vi "Field Draw Robots.vi"(3 "Draw Targets?":T1, 4 "RobotRef":refnum<class "Robot.lvclass">[](array[class]), 5 "Draw Number":bool=TRUE, 6 "color(black)":u32, 8 "Picture In":picture, 9 "Offset":cluster{"Width":dbl, "Height":dbl}, 10 "Scale":dbl, 11 "color":enum16{"Azul", "Amarelo"}(ring)) -> (0 "Picture Out":picture, 1 "Offset Out":cluster{"Width":dbl, "Height":dbl}, 2 "Scale Out":dbl)   [LabVIEW 2018]
uses:
  DrawTargets.ctl
  Robot_class/Robot.lvclass
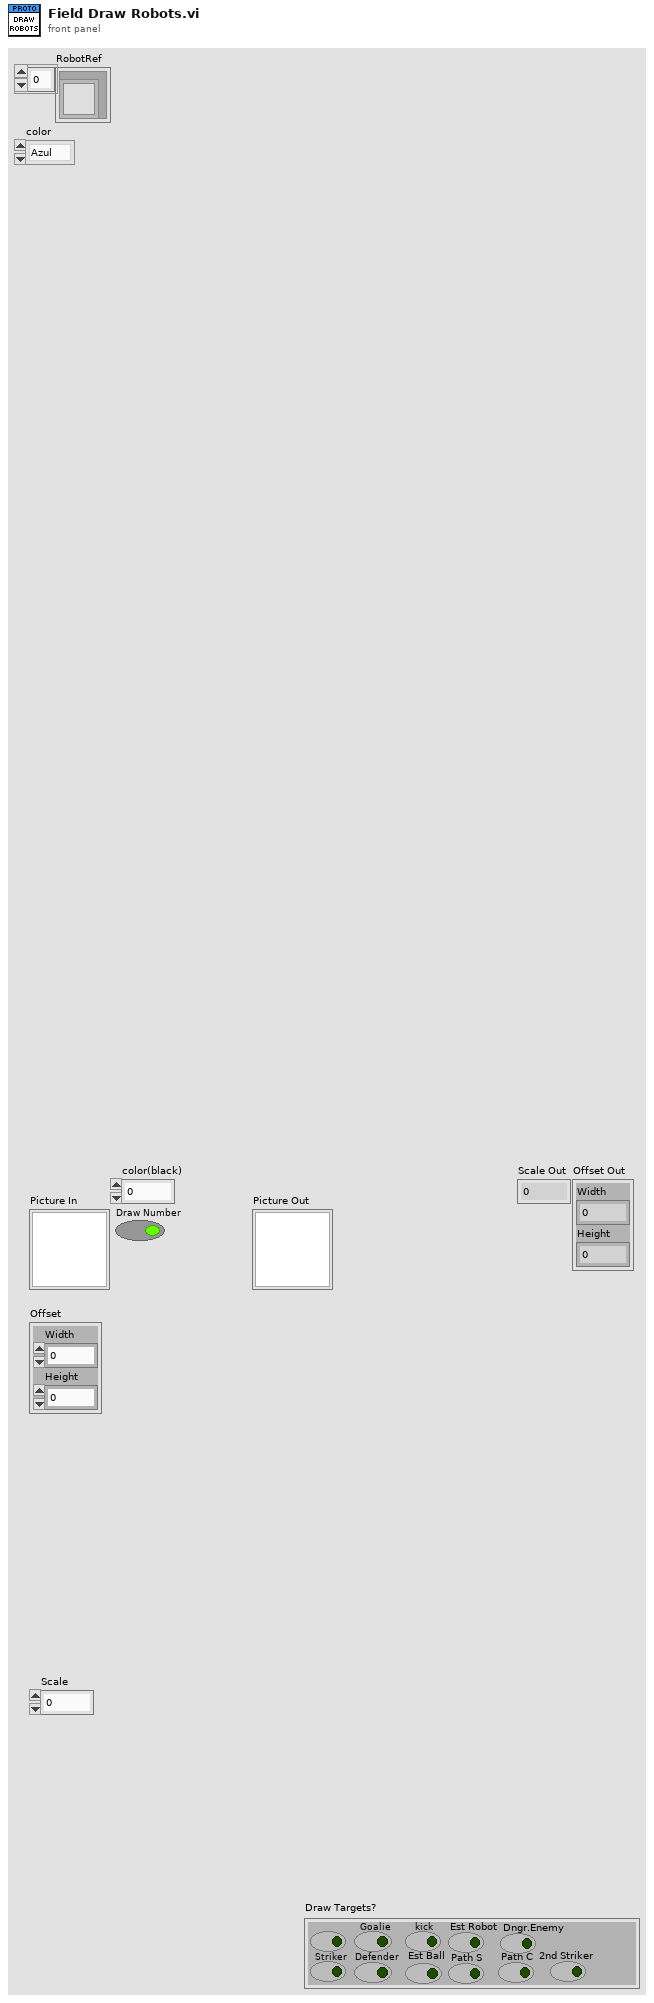
[diagram p1: front panel]
types:
  T1 = typedef "DrawTargets.ctl" = cluster{"Attacker":bool, "Striker":bool, "Goalie":bool, "Defender":bool, "kick":bool, "Est Ball":bool, "Est Robot":bool, "Path S":bool, "Path C":bool, "Dngr.Enemy":bool, "2nd Striker":bool}
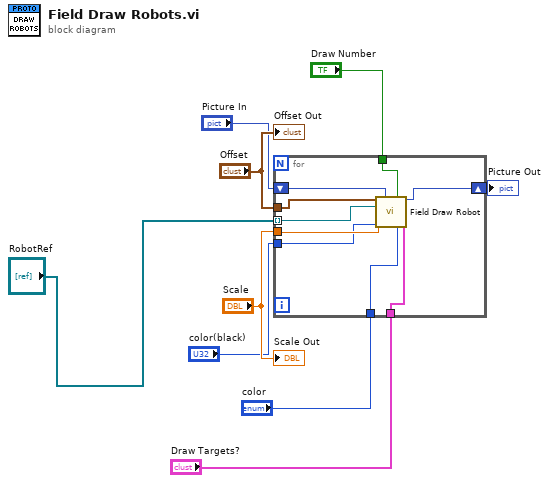
[diagram p0: block diagram]
diagram:
  n1 = for {
    tunnel: "Scale" -> [w14]
    tunnel: "Offset" -> [w15]
    shift-right: [w18] -> w5
    shift-left: "Picture In" -> [w16]
    tunnel: "color(black)" -> [w13]
    tunnel: "Draw Number" -> [w17]
    tunnel: "Draw Targets?" -> [w12]
    tunnel: "RobotRef" -> [w11] mode=indexing
    tunnel: "color" -> [w10]
    n2 = call "Field Draw Robot.vi"("Offset"=w15, "picture in"=w16, "Draw Number"=w17, "Robot"=w11, "Scale mm/pixel"=w14, "color(black)"=w13, "color"=w10, "Draw Targets?"=w12) -> ("picture out"=w18:picture)  [unwired: 7 in]
  }
  "Picture Out" <- w5
  "Scale Out" <- "Scale"
  "Offset Out" <- "Offset"
